vi "Detect Keystroke.vi"(4 "PlatMods":T2, 5 "ScanCode":i16) -> (1 "Keystroke":T1)   [LabVIEW 2011]
uses:
  Keystroke.ctl
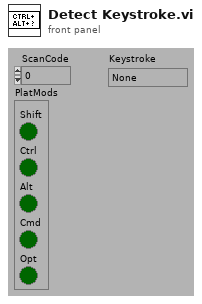
[diagram p1: front panel]
types:
  T1 = typedef "Keystroke.ctl" = enum16{"None", "CTRL+ALT+A", "CTRL+ALT+F", "CTRL+ALT+L", "CTRL+ALT+M", "CTRL+ALT+P", "CTRL+ALT+R"}
  T2 = cluster{"Shift":bool, "Ctrl":bool, "Alt":bool, "Cmd":bool, "Opt":bool}
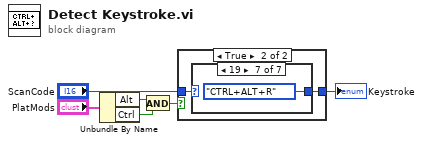
[diagram p0: block diagram]
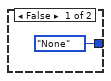
[diagram p2: hidden frame]
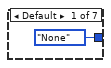
[diagram p3: hidden frame]
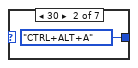
[diagram p4: hidden frame]
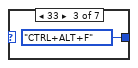
[diagram p5: hidden frame]
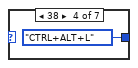
[diagram p6: hidden frame]
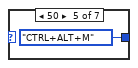
[diagram p7: hidden frame]
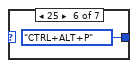
[diagram p8: hidden frame]
diagram:
  n1 = Unbundle By Name("PlatMods") -> ("Alt"=w5:bool, "Ctrl"=w4:bool)
  n2 = And(x=w5, y=w4) -> (x .and. y?=w3:bool)
  n3 = case shown="True" w3 {
    tunnel: "ScanCode" -> [_ w9]
    tunnel: [Keystroke."None" ("Keystroke") w8] -> w1
    frame False {
    }
    frame True {
      n4 = case shown="19" w9 {
        tunnel: [Keystroke."None" ("Keystroke") Keystroke."CTRL+ALT+A" ("Keystroke") Keystroke."CTRL+ALT+F" ("Keystroke") Keystroke."CTRL+ALT+L" ("Keystroke") Keystroke."CTRL+ALT+M" ("Keystroke") Keystroke."CTRL+ALT+P" ("Keystroke") Keystroke."CTRL+ALT+R" ("Keystroke")] -> w8
        frame Default {
        }
        frame 30 {
        }
        frame 33 {
        }
        frame 38 {
        }
        frame 50 {
        }
        frame 25 {
        }
        frame 19 {
        }
      }
    }
  }
  "Keystroke" <- w1
